vi "Generic Controller with DSA.vi"() -> ()   [LabVIEW 2017]
uses:
  <vilib>/myRIO/Instrument Drivers/Onboard IO/AO/typedefs/AO Reference.ctl
  <vilib>/myRIO/Common/Instrument Driver Framework/Utilities/typedefs/myRIO Generic Hardware Reference.ctl
  <vilib>/myRIO/Common/Instrument Driver Framework/Utilities/typedefs/Hardware Version Enum.ctl
  <vilib>/myRIO/Common/Instrument Driver Framework/Utilities/typedefs/myRIO v1.0 Reference.ctl
  <vilib>/myRIO/Common/Instrument Driver Framework/Utilities/typedefs/Generic FPGA Reference.ctl
  <vilib>/myRIO/Common/Instrument Driver Framework/myRIO v1.0/AO/typedefs/AO Channels List.ctl
  <vilib>/myRIO/Common/Instrument Driver Framework/myRIO v1.0/AO/typedefs/AO Channels Enum.ctl
  <vilib>/myRIO/Common/Instrument Driver Framework/Utilities/typedefs/Analog Scaling Constants List.ctl
  <vilib>/myRIO/Common/Instrument Driver Framework/Utilities/typedefs/Analog Scaling Constants.ctl
  <vilib>/userdefined/High Color/nirio_resource_hc.ctl
  <vilib>/Simulation/Scripting/Companion Diagram/SimConfigNode/SimParams.ctl
  <vilib>/Simulation/Scripting/Companion Diagram/SimConfigNode/_simSolvers.ctl
  <vilib>/Simulation/Implementation/Shared/SIMSCR Execution Mode.ctl
  <vilib>/Platform/TimedLoop/XDataNode/timing_clust.ctl
  <vilib>/Platform/TimedLoop/XDataNode/nitl_modes.ctl
  <vilib>/Platform/TimedLoop/XDataNode/wakeup.ctl
  <vilib>/Simulation/Param Hierarchy/Typedefs/SIMPH Param Control Actions.ctl
  <vilib>/Simulation/Implementation/Shared/SIM limit type.ctl
  <vilib>/Simulation/Scripting/Editor Utilities/SIM subVI tag data.ctl
  <vilib>/Simulation/Scripting/Editor Utilities/SIM subVI execution type.ctl
  <vilib>/myRIO/Instrument Drivers/Onboard IO/AI/typedefs/AI Reference.ctl
  <vilib>/myRIO/Common/Instrument Driver Framework/myRIO v1.0/AI/typedefs/AI Channels List.ctl
  <vilib>/myRIO/Common/Instrument Driver Framework/myRIO v1.0/AI/typedefs/AI Channels Enum.ctl
  <vilib>/myRIO/Common/Instrument Driver Framework/Utilities/vis/Is FPGA Ref Available.vi
  <vilib>/myRIO/Common/Instrument Driver Framework/myRIO v1.0/AO/vis/myRIO v1.1 Open AO.vi
  <vilib>/myRIO/Instrument Drivers/Onboard IO/AO/vis/Write.vi
  <vilib>/Simulation/Implementation/Shared/NILVSim_ParamChanged.vi
  <vilib>/Simulation/Implementation/Shared/NILVSim_FinishedLate.vi
  <vilib>/Simulation/Implementation/Shared/NILVSIM_BeginStep.vi
  <vilib>/myRIO/Common/Instrument Driver Framework/myRIO v1.0/AI/vis/myRIO v1.1 Open AI.vi
  <vilib>/myRIO/Instrument Drivers/Onboard IO/AI/vis/Read.vi
  <vilib>/Simulation/Utility/Implementation/SIM Halt.vi
  <vilib>/Simulation/DataSources/Implementation/NILVSim Signal Generator.llb/SIM Signal Generator (scalar).vi
  <vilib>/Simulation/Utility/Implementation/SIM SimulationParams.vi
  <vilib>/Simulation/ContinuousLinear/Implementation/NILVSim Integrator new.llb/SIM Integrator distributor (scalar).vi
  <vilib>/Simulation/Implementation/Shared/SIM Is Init or Final Stage.vi
  <vilib>/Simulation/Implementation/Shared/SIM Fire Discrete SubVI.vi
  <vilib>/Simulation/SignalArithmetic/Implementation/NILVSim Gain.llb/SIM Gain (scalar).vi
  <vilib>/Simulation/ContinuousLinear/Implementation/NILVSim Integrator new.llb/SIM Integrator collector (scalar).vi
  <vilib>/Simulation/ContinuousLinear/Implementation/NILVSim Transfer Function Direct.llb/SIM Transfer Function Direct (SISO).vi
  <vilib>/Simulation/Implementation/Shared/NILVSim_Manager.vi
  <vilib>/Utility/error.llb/Clear Errors.vi
  <vilib>/Simulation/Implementation/Shared/NILVSim_FinalizeModel.vi
  <vilib>/myRIO/Common/Instrument Driver Framework/Utilities/vis/Validate Channels.vi
  <vilib>/myRIO/Common/Instrument Driver Framework/myRIO v1.0/AO/vis/myRIO v1.0 Reserve AO.vi
  <vilib>/myRIO/Common/Instrument Driver Framework/myRIO v1.0/AI/vis/myRIO v1.0 Reserve AI.vi
  <vilib>/Simulation/Utility/Implementation/NILVSim SimulationParams (core).vi
  <vilib>/Simulation/Implementation/Shared/SIM Fire Discrete SubVI (Core).vi
  <vilib>/myRIO/Common/Instrument Driver Framework/myRIO v1.0/AO/vis/myRIO v1.0 Build MUX Configuration AO.vi
  <vilib>/myRIO/Common/Instrument Driver Framework/myRIO v1.0/Resource Manager/vis/myRIO v1.0 Reserve Channel List.vi
  <vilib>/myRIO/Common/Instrument Driver Framework/myRIO v1.0/AI/vis/myRIO v1.0 Build MUX Configuration AI.vi
  <vilib>/myRIO/Common/Instrument Driver Framework/myRIO v1.0/Resource Manager/vis/myRIO v1.0 Reserve Channel.vi
  <vilib>/myRIO/Common/Instrument Driver Framework/myRIO v1.0/Resource Manager/vis/myRIO v1.0 Unreserve Channel.vi
  <vilib>/myRIO/Common/Instrument Driver Framework/myRIO v1.0/Resource Manager/vis/myRIO v1.0 Build Mutex Name.vi
  <vilib>/Utility/VariantDataType/GetNumericInfo.vi
  <vilib>/Utility/error.llb/Error Cluster From Error Code.vi
  <vilib>/myRIO/Common/Instrument Driver Framework/myRIO v1.0/myRIO v1.1 Open.vi
  <vilib>/myRIO/Common/Instrument Driver Framework/myRIO v1.0/AO/vis/myRIO v1.0 Get Scaling Constants AO.vi
  <vilib>/myRIO/Common/Instrument Driver Framework/Utilities/vis/IO Manager.vi
  <vilib>/myRIO/Common/Instrument Driver Framework/Utilities/vis/Configuration Manager.vi
  <vilib>/myRIO/Common/Instrument Driver Framework/myRIO v1.0/myRIO v1.0 Close.vi
  <vilib>/myRIO/Common/Instrument Driver Framework/myRIO v1.0/AO/vis/myRIO v1.0 Write AO.vi
  <vilib>/Simulation/Implementation/Shared/SIM Unbundle Sim Info.vi
  <vilib>/Simulation/Implementation/Shared/SIMSH Read Queue.vi
  <vilib>/Simulation/Implementation/Shared/NILVSim_Initialize.vi
  <vilib>/myRIO/Common/Instrument Driver Framework/myRIO v1.0/AI/vis/myRIO v1.0 Get Scaling Constants AI.vi
  <vilib>/myRIO/Common/Instrument Driver Framework/myRIO v1.0/AI/vis/myRIO v1.0 Read AI.vi
  <vilib>/Simulation/Utility/Implementation/NILVSim Get Time and IsAcceptedStep.vi
  <vilib>/Simulation/Implementation/Shared/NILVSim_GetModelError.vi
  <vilib>/Simulation/Implementation/Shared/SIM Bundle Sim Info.vi
  <vilib>/myRIO/Express VI/Onboard IO/AO/AO Express VI.xnode
  <vilib>/myRIO/Instrument Drivers/Onboard IO/AO/vis/myRIO AO Open.xnode
  <vilib>/Platform/TimedLoop/XDataNode/XDataNode.xnode
  <vilib>/Simulation/Scripting/Companion Diagram/SimConfigNode/SimDog.xnode
  <vilib>/myRIO/Express VI/Onboard IO/AI/AI Express VI.xnode
  <vilib>/myRIO/Instrument Drivers/Onboard IO/AI/vis/myRIO AI Open.xnode
  <vilib>/Simulation/Implementation/XNodeFramework/SimXNode/SimX.xnode
  <vilib>/Simulation/ContinuousLinear/Implementation/NILVSim Integrator new.llb/SIM Integrator (scalar).vi
  <vilib>/myRIO/Instrument Drivers/Onboard IO/AO/AO.lvlib
  <vilib>/Platform/TimedLoop/XDataNode/XDNodeRunTimeDep.lvlib
  <vilib>/myRIO/Instrument Drivers/Onboard IO/AI/AI.lvlib
  <vilib>/Simulation/Implementation/Shared/NI_SIM_Implementation.lvlib
panel:
  in  "Tab Control":T1(tab)
  in  "alpha":dbl=10.0
  in  "Td":dbl=0.0025
  in  "ON? 2":bool=TRUE
  in  "Upper":dbl=10.0
  in  "Lower":dbl=-10.0
  in  "Ti":dbl=0.0032
  in  "ON?":bool
  in  "Kp":dbl=-6.1
  in  "Feedback?":bool=TRUE
  in  "Amplitude":dbl
  in  "Frequency":dbl=6.0
  in  "Offset":dbl=0.04
  in  "Signal Type":u16(ring) items=["Sine", "Square", "Sawtooth", "Random"]
  in  "Control Time Step [s]":dbl=0.0005
  out "Control Loop Execution Time [us]":u32=249
  out "Control Loop Late Cycles":i32=4
  in  "External Reference?":bool
  in  "Internal Reference?":bool
  out "Oscilliscope":T2(graph)={"Double"=0.0, "Double"=-0.429687544, "Double"=-2.605132217660948}
  out "Plot Loop Execution Time [us]":u32=565
  in  "TLP":dbl=0.0016
  in  "ON? 3":bool=TRUE
  out "DSA Loop Late Cycles":i32
  out "DSA Loop Execution Time (us)":u32=518
  out "Bode Phase":cluster{dbl[], dbl[]}(graph)={[0.5, 0.5413183669370273, 0.5860511487667401, 0.6344805015839611, 0.6869118979416314, 0.7436760536467557, 0.8051310137804697, 0.8716644110999939, 0.9436959110675486, 1.021679858928471, 1.1061081455352246, 1.1975133099937427, 1.2964718987023336, 1.4036081019705886, 1.5195976911565985, 1.6451722811563343, 1.781123945131221, 1.9283102105817356, 2.0876594682802008, 2.2601768281801213, 2.446950459238747, 2.649158453141854, 2.8680762552243393, 3.1050847094578082, 3.3616787682496687, 3.6394769219915744, 3.9402314078349554, 4.265839262086405, 4.618354285936929, 5.0], [1.1113686665475342, -3.3715278086255864, -4.589885860566625, 4.2977168391159495, -5.935917889942033, -4.065647863471284, -1.6158442409451226, 89.88669974540309, 70.62051910594798, 85.09208365468596, 77.00702996239605, 43.46670720052916, -2.679772948914234, -13.624983803961307, -15.540260691171454, 92.75050103936908, 65.66683642318564, 75.45823036346658, -6.144982127247204, -15.535633497005172, 63.51301466180453, -63.682873216459825, 64.9522046090478, -8.82711887868328, 21.07479668472711, 17.564687083801523, -3.3971444036905964, -1.5249224157625818, -0.7028110405561847, -10.27143238102737]}
  out "Bode Magnitude":cluster{dbl[], dbl[]}(graph)={[0.5, 0.5413183669370273, 0.5860511487667401, 0.6344805015839611, 0.6869118979416314, 0.7436760536467557, 0.8051310137804697, 0.8716644110999939, 0.9436959110675486, 1.021679858928471, 1.1061081455352246, 1.1975133099937427, 1.2964718987023336, 1.4036081019705886, 1.5195976911565985, 1.6451722811563343, 1.781123945131221, 1.9283102105817356, 2.0876594682802008, 2.2601768281801213, 2.446950459238747, 2.649158453141854, 2.8680762552243393, 3.1050847094578082, 3.3616787682496687, 3.6394769219915744, 3.9402314078349554, 4.265839262086405, 4.618354285936929, 5.0], [0.1705227721348142, 0.1544347188687134, 0.17822285984429972, 0.14890848479663207, 0.1556998177366923, 0.14229088999240103, 0.16278672493894716, 0.003754159491098782, 0.007278718638241219, 0.004240175333076675, 0.006838804760208183, 0.0620848402718586, 0.2688203440065051, 0.18402355770794834, 0.14230747948833408, 0.0022001806117035714, 0.003041606136419923, 0.004363980185748692, 0.14874482575873157, 0.16349358042061182, 0.014255687186903598, 0.18481000781841925, 0.01857244313127678, 0.16431673209279352, 0.212603582029145, 0.27808950044049247, 0.29698413361699644, 0.28891790694466224, 0.2871852670976697, 0.29582840306665104]}
  in  "START":bool
  out "Running":bool
  in  "Excitation Specs":T3={"Initial Frequency"=0.5, "Final Frequency"=5.0, "Number of Frequencies"=30, "DSA Samping Time [s]"=0.0005, "Amplitude"=0.01, "Offset"=0.0, "Freq Unit"=TRUE}
  in  "Cycle Specs":T4={"Cycles To Settle (M)"=1, "Cycles To Calculate (N)"=10}
  out "Stopped":bool=TRUE
  in  "STOP":bool
  out "Live Signals":cluster{"DSA Excitation":dbl, "output y(t)":dbl}(graph)={"DSA Excitation"=-2.605132217660948, "output y(t)"=-0.429687544}
  in  "Exit Program":bool
  # "PMCL Generic Controller with DSA"
  # "Control Loop Parameters"
  # "Reference Signal"
  # "Internal Reference"
  # "Controllers"
  # "Controllers Implemenetation"
  # "The Lead-Lag Controller has the form:"
  # "HF LP\nFilter:"
  # "Proportional:"
  # "Intergrator Limits"
  # "Lag:"
  # "Note: Ti is the integrator time constant. Ti = 1/Ki"
  # "Lead:"
  # "Note: Td is the lag compensator time constant."
  # "Note: Both references should be off when running the DSA!"
  # "Dynamic Signal Analyzer"
  # "Controls"
  # "Phase"
  # "Magnitude"
  # "Excitation Frequencies"
  # "Excitation Magnitude"
  # "Freq. Units"
  # "[Hz]"
  # "[rad/s]"
  # "Using the Controller\n \n(1) Press CNTRL + E to pull up the back pannel code.\n\n(2) Program your controller into the area labed:  \n\n(3) Check                             to enable your controller."
  # "Closed Loop Controller"
  # "Wiring Details\n  \n       - AO 0:   Control Effort\n \n       - AI   0+: Plant / Sensor Ouput\n       - AI   0- : AGND\n \n       - AI   1+: External Signal Generator \n       - AI   1- : AGND"
  # "- Ideally you would want AI 0+ to be the plant output. However as the plant output is not \n         always a voltage, this will often be a sensor output. As a result, the measured frequency \n         response (bode plots) will be gained by the gain of the sensor.\n \n              ~ Usually the gain of the sensor is a constant though so just divide the magnitude by it."
  # "Using the DSA\n \n(1) Press CNTRL + E to pull up the back pannel code.\n\n(2) Rewire                                        and                                        according to the TF you want to measure. See DSA Theory Tab for help.\n \n         TF = (DSA CH B) / (DSA CH B)  \n \n      - If using the DSA to measure a TF that's apart of the closed loop, make sure the closed loop is stable &                               .      \n \n(3) Turn off the reference signals:                                             &\n\n      - If using one of the reference signals to instead provide a DC bias, simply turn the amplitude to zero intead.\n\n(4) Set the DSA Excitation Specs & Cycel Specs: \n \n      - Inital Frequency: First frequnecy we want to measure. Typically atleast 1 decade before frequency of interest\n \n      - Final Frequency: Final frequency we want to measure. Typically atleast 1 decade beyond frequency of interest\n  \n             ~ Note:  Max Final Frequency = Sampling Rate/2     as this is out Nyquist Frequency          \n \n      - Number of Frequnecies: Something reasonable like 30 frequencies every decade measured\n \n      - Amplitude: Largest Amplitude such that the control effort does not staturate\n \n      - Cycles to Settle (M): 1 minimum for low frequencies (below 5 Hz) & 10 minimum for high frequencies (above 100 Hz)\n \n      - Cycles to Calculate (N): 1 minimum for low frequencies (below 5 Hz) & 100 minimum for high frequencies (above 100 Hz)  \n \n      * TO MAKE THE DSA FASTER WITH BETTER RESULTS, RUN THE DSA MULTIPLE TIMES!!! \n         ex. from     0.5 Hz - 5 Hz w/ M =1,    N =1, 5 Hz - 50 Hz w/ M = 1,  N = 10,     &    50 Hz - 500 Hz w/ M = 10, N = 100 \n \n(5) Press START to start the DSA.\n\n(6) Press STOP to stop the DSA if needed or it will stop when it is finished."
  # "Running the Program\n \n(1) Set the Controller Time Step, the rate at which the myRIO samples the sensor and updates the control effort sent to the plant.\n      This is located on the on the Controller Tab.\n\n      - Controller Loop Rate = 1/(Controller Time Step)     where the default is 0.001 sec which is a sampling rate of 1 kHz.\n \n      - If the Control Loop Late Cycles indicator rapidly increases, the control loop needs to run at a slower rate.\n \n      - If you update the Controller Time Step, exist and rerun the program! This must be set before the program starts.\n\n(2) If you plan on using the Dynamics Signal Anayzer to measure a frequency response, set the DSA Sampling Time [s], the rate at \n      which the dynamic signal analyzer samples the control signals at. This is located on the on the DSA Tab.\n\n      - DSA Sampling Rate = 1/(DSA Sampling Time)     where the default is 0.001 sec which is a sampling rate of 1 kHz.\n\n      - Typically, the  DSA Sampling Time =  Controller Time Step.\n \n      - Note: If the DSA Loop Late Cycles indicator rapidly increases, the DSA loop needs to run at a slower rate.\n \n      - If you update the Controller Sampling Time, exist and rerun the program! This must be set before the program starts.\n \n \n(2) Press the white arrow above,          , to start the program.\n \n(3) Use the program. See Using the Controller, Using the DSA, and/or Collecting Data.\n \n(4)  Click EXIT PROGRAM in the upper right hand corner to stop the progam. \n\n      - NEVER CLICK the small stop sign,          , unless it's an emergency as this will not reset your AOs to zero."
  # "Collecting Data\n \n(1) Right click the graph and select Export.\n \n      - NOTE: You can only record what is shown on the graph!\n\n(2) Choose the format you want to export your data to:\n \n       - Export Data To Clipboard: Copies it so you can paste it into a program like Excel, Matlab, Notepad, etc.\n \n       - Export Data To Excel: Opens up your data in Excel.\n \n       - Export Simpliefed Image... : Saves your data as a cleaned up screenshot picture\n  \n Changing the Total Time of Data Recorded\n \nTo change the length of time displayed on the graph and thus the length of time you record data for, right click and select Chart History Length while the porgram is NOT running. \n \n        Chart History Length = [ (Desired Length of Time in Sec) / (Controller Time Step) ] + 1\n \n        * The + 1 is necessary to prevent the axes from drifting as LabVIEW includes both the start and final sample in the total time.\n\nThen double click on the starting and final tick of the time axis. Type a new a time into each tick such that the total time elapsed between the two ticks is your desired length of time to be displayed."
  # "A DSA, or Dynamic Signal Analyzer is a tool that measures a the frequency response of a transfer function and plots its corresponding bode plots."
  # "A DSA works in 3 steps:\n\n      (1) The DSA  inputs a swept sine wave (a sine wave that increaes in frequency), D, into the control loop. Here the swept sine wave is being added to the reference at the feedback summing junction. The swept sine wave will show up through out the control loop with different a \n            magnitude and phase at each of its frequencies. How the magnitude and phase of this swept sine wave changes at each frequency through out the control loop is what we care about.\n\n      (2) Then the DSA measures the swept sine wave at two points through out the control loop.\n\n      (3) Finally the DSA finds the frequency response of the  transfer function between the two points measured. This is visually shown as a bode plot. \n            \n                  - The  magnitude of the frequency response is the magnitude of the swept sine wave measured at the first point divided the  magnitude of the swept sine wave measured at the second point. \n\n                  - The phase of the frequency response is the phase of the swept sine wave measured at the first point minus the phase of the swept sine wave measured at the second point.\n\nThree transfer functions we often care about are the plant P, return ratio RR, and the closed loop CL. Thus below we will go through how to measure the frequency response of those with the DSA.\n\n      - Plant: The plant is just the ratio of the output of the plant to its input, P = Y/C. Thus the DSA finds the frequency response of the plant by measuring the signal output by the plant (a swept sine wave), Y, and the signal input to the plant (a swept sine wave), C. Then it divides \n                    the magnitude of Y by the magnitude of C and subtracts the phase of C from the phase of Y at each frequency of the swept sine wave. This provides the frequency reponse of the plant as it changes with freqency.\n\n      - Return Ratio: The return ratio is just the ratio of the output of the loop to its input, RR = M/E. Thus the DSA finds the frequency response of the return ratio by measuring the signal output by the loop (a swept sine wave), M, and the signal input to the loop (a swept sine wave), E. \n                                 Then it divides the magnitude of M by the magnitude of E and subtracts the phase of E from the phase of M at each frequency of the swept sine wave. This provides the frequency reponse of the return ratio as it changes with freqency.\n\n      - Closed Loop: The closed loop is just the ratio of the output of the closed loop to its input, CL = Y/D. Thus the DSA finds the frequency response of the closed loop by measuring the signal output by the closed loop (a swept sine  wave), Y, and the signal input to the closed loop \n                                 (a swept sine wave), D. Then it divides the magnitude of Y by the magnitude of D and subtracts the phase of R from the phase of Y at each frequency of the swept sine wave. This provides the frequency reponse of the closed loop as it changes with freqency."
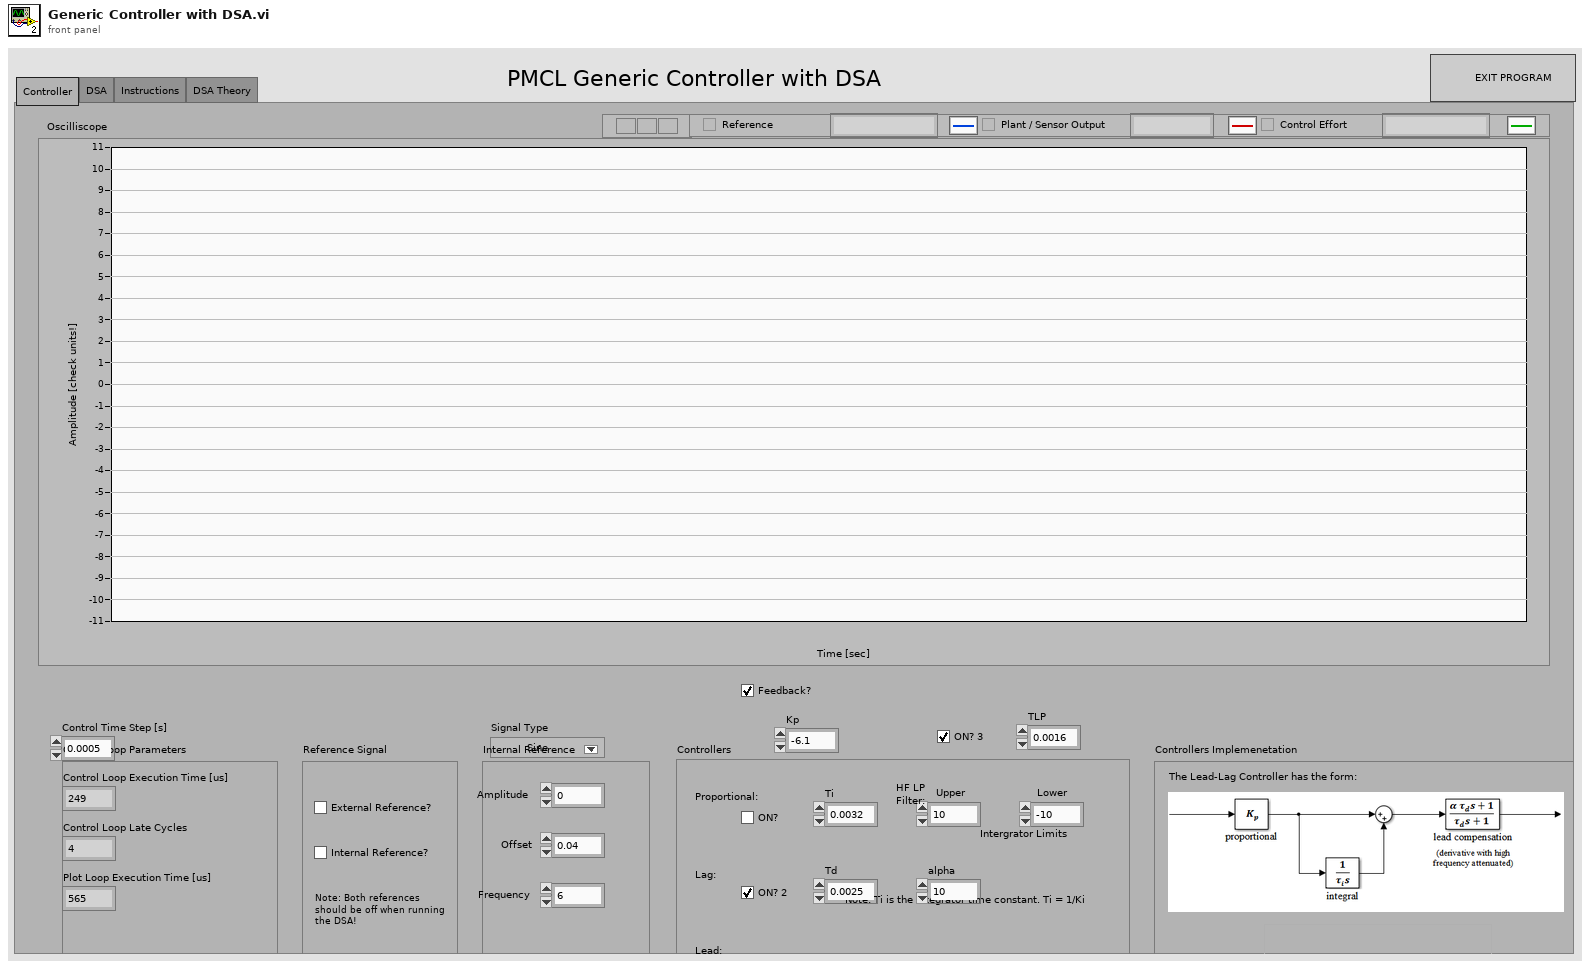
[diagram p1: front panel]
types:
  T1 = enum32{"Controller", "DSA", "Instructions", "DSA Theory"}
  T2 = cluster{"Double":dbl, "Double":dbl, "Double":dbl}
  T3 = cluster{"Initial Frequency":dbl, "Final Frequency":dbl, "Number of Frequencies":i16, "DSA Samping Time [s]":dbl, "Amplitude":dbl, "Offset":dbl, "Freq Unit":bool}
  T4 = cluster{"Cycles To Settle (M)":i16, "Cycles To Calculate (N)":i16}
  T5 = cluster{"DSA Excitation":dbl, "output y(t)":dbl}[]
  T6 = cluster{"Double":dbl, "Double":dbl, "Double":dbl}[]
  T7 = typedef "AO.lvlib/AO Reference.ctl" = cluster{"myRIO Reference":T8, "AO Channel List":T12, "AO Scaling Constant List":T14}
  T8 = typedef "myRIO Generic Hardware Reference.ctl" = cluster{"myRIO Model":T9, "myRIO Hardware Reference":T10}
  T9 = typedef "Hardware Version Enum.ctl" = enum16{"Unknown", "myRIO-1900", "myRIO-1950", "roboRIO", "NI ELVIS RIO CM"}
  T10 = typedef "myRIO v1.0 Reference.ctl" = cluster{"Generic FPGA Reference":T11, "Allow multiple opens":bool}
  T11 = typedef "Generic FPGA Reference.ctl" = refnum<k20>
  T12 = typedef "AO Channels List.ctl" = T13[]
  T13 = typedef "AO Channels Enum.ctl" = enum16{"Not Connected", "AudioOut/Left", "AudioOut/Right", "C/AO0", "C/AO1", "A/AO0", "A/AO1", "B/AO0", "B/AO1"}
  T14 = typedef "Analog Scaling Constants List.ctl" = T15[]
  T15 = typedef "Analog Scaling Constants.ctl" = cluster{"LSB Weight (Volts)":dbl, "Offset (Volts)":dbl, "Signed?":bool}
  T16 = typedef "nirio_resource_hc.ctl" = tag
  T17 = typedef "XDNodeRunTimeDep.lvlib/timing_clust.ctl" = cluster{"Expected End [f-1]":u64, "Actual End [f-1]":u64, "Finished Late? [f-1]":bool, "Expected End [i-1]":u64, "Actual End [i-1]":u64, "Finished Late? [i-1]":bool, "Expected Start [i]":u64, "Actual Start [i]":u64, "Expected Start [f]":u64, "Actual Start [f]":u64, "Source Name":string, "Structure Name":string, "Period":i64, "Deadline":i64, "Offset":i64, "Start":i64, "Priority":i32, "Timeout":i32, "Mode":T18, "Wakeup Reason":T19, "Error":errorcluster, "Source Type":string, "Secondary Source Type":string, "Global End Time":u64, "Global Start Time":u64, "Frame Duration":u64, "Iteration Duration":u64, "Assigned CPU":i32, "I/O Scan Engine Mode":u32}
  T18 = typedef "XDNodeRunTimeDep.lvlib/nitl_modes.ctl" = enum32{"No Change", "Process missed periods, maintain original phase", "Discard missed periods, maintain original phase", "Process missed periods, ignore original phase", "Discard missed periods, ignore original phase"}
  T19 = typedef "XDNodeRunTimeDep.lvlib/wakeup.ctl" = enum32{"Normal", "Aborted", "Asynchronous wakeup", "Timing source error", "Timed loop error", "Timeout"}
  T20 = typedef "SimParams.ctl" = cluster{"Initial Time (s)":dbl, "Final Time (s)":dbl, "Step Size (s)":dbl, "ODE Solver":T21, "Minimum Step Size (s)":dbl, "Maximum Step Size (s)":dbl, "Relative Tolerance":dbl, "Absolute Tolerance":dbl, "Software Timing":bool, "Initial Step Size (s)":dbl, "Automatic Fixed Step Size?":bool, "Automatic Discrete Step Size?":bool, "Discrete Step Size (s)":dbl, "Calculate using Time Step":bool, "Solver Wired?":bool, "Prev.Frm.Expected End":u64, "Prev.Frm.Actual End":u64, "Prev.Frm.Finished Late?":bool, "Prev.Iter.Expected End":u64, "Prev.Iter.Actual End":u64, "Prev.Iter.Finished Late?":bool, "Expected Iteration Start":u64, "Actual Iteration Start":u64, "Expected Frame Start":u64, "Actual Frame Start":u64, "Source Name":string, "Name":string, "Period":i64, "Deadline":i64, "Offset":i64, "Start":i64, "Priority":i32, "Timeout":i32, "Processor":i32, "Mode":enum32{"No Change", "Process missed periods, maintain original phase", "Discard missed periods, maintain original phase", "Process missed periods, ignore original phase", "Discard missed periods, ignore original phase"}, "Wakeup reason":enum32{"Normal", "Aborted", "Asynchronous wakeup", "Timing source error", "Timed loop error", "Timeout"}, "Error":errorcluster, "Source Type":string, "Secondary Source Type":string, "Global End Time":u64, "Global Start Time":u64, "Full Solver Reset":bool, "Execution Mode":T22, "Nan/Inf Check":bool, "Custom Solver Library":string, "Solver Is Variable":bool, "custom solver name":string, "Signal Collection Decimation":u32}
  T21 = typedef "_simSolvers.ctl" = enum16{"Runge-Kutta 1 (Euler)", "Runge-Kutta 2", "Runge-Kutta 3", "Runge-Kutta 4", "Runge-Kutta 23 (variable)", "Runge-Kutta 45 (variable)", "BDF (variable)", "Adams-Moulton (variable)", "Rosenbrock (variable)", "Discrete States Only", "SDIRK 4 (variable)", "Radau 5 (variable)", "Radau 9 (variable)", "Radau 13 (variable)", "Radau [Variable Order] (variable)", "Gear's Method (variable)", "Linearizer", "State Query", "Trim Eval", "Custom Solver"}
  T22 = typedef "SIMSCR Execution Mode.ctl" = enum16{"Simulate to Completion", "Single Time-Step Simulation (Fixed Step Only)"}
  T23 = typedef "AI.lvlib/AI Reference.ctl" = cluster{"myRIO Reference":T8, "AI Channels List":T24, "AI Scaling Constants List":T14}
  T24 = typedef "AI Channels List.ctl" = T25[]
  T25 = typedef "AI Channels Enum.ctl" = enum16{"Not Connected", "AudioIn/Left", "AudioIn/Right", "C/AI0", "C/AI1", "A/AI0", "A/AI1", "A/AI2", "A/AI3", "B/AI0", "B/AI1", "B/AI2", "B/AI3", "AI/AI0", "AI/AI1", "AI/AI2", "AI/AI3"}
  T26 = typedef "SIMPH Param Control Actions.ctl" = enum16{"get params", "set params"}
  T27 = typedef "SIM subVI tag data.ctl" = cluster{"period":dbl, "skew":dbl, "Simulation execution type":T28}
  T28 = typedef "SIM subVI execution type.ctl" = enum16{"Function call", "Discrete", "Continuous", "Initialization only", "Final step only"}
  T29 = typedef "SIM limit type.ctl" = enum16{"upper", "lower", "both", "none"}
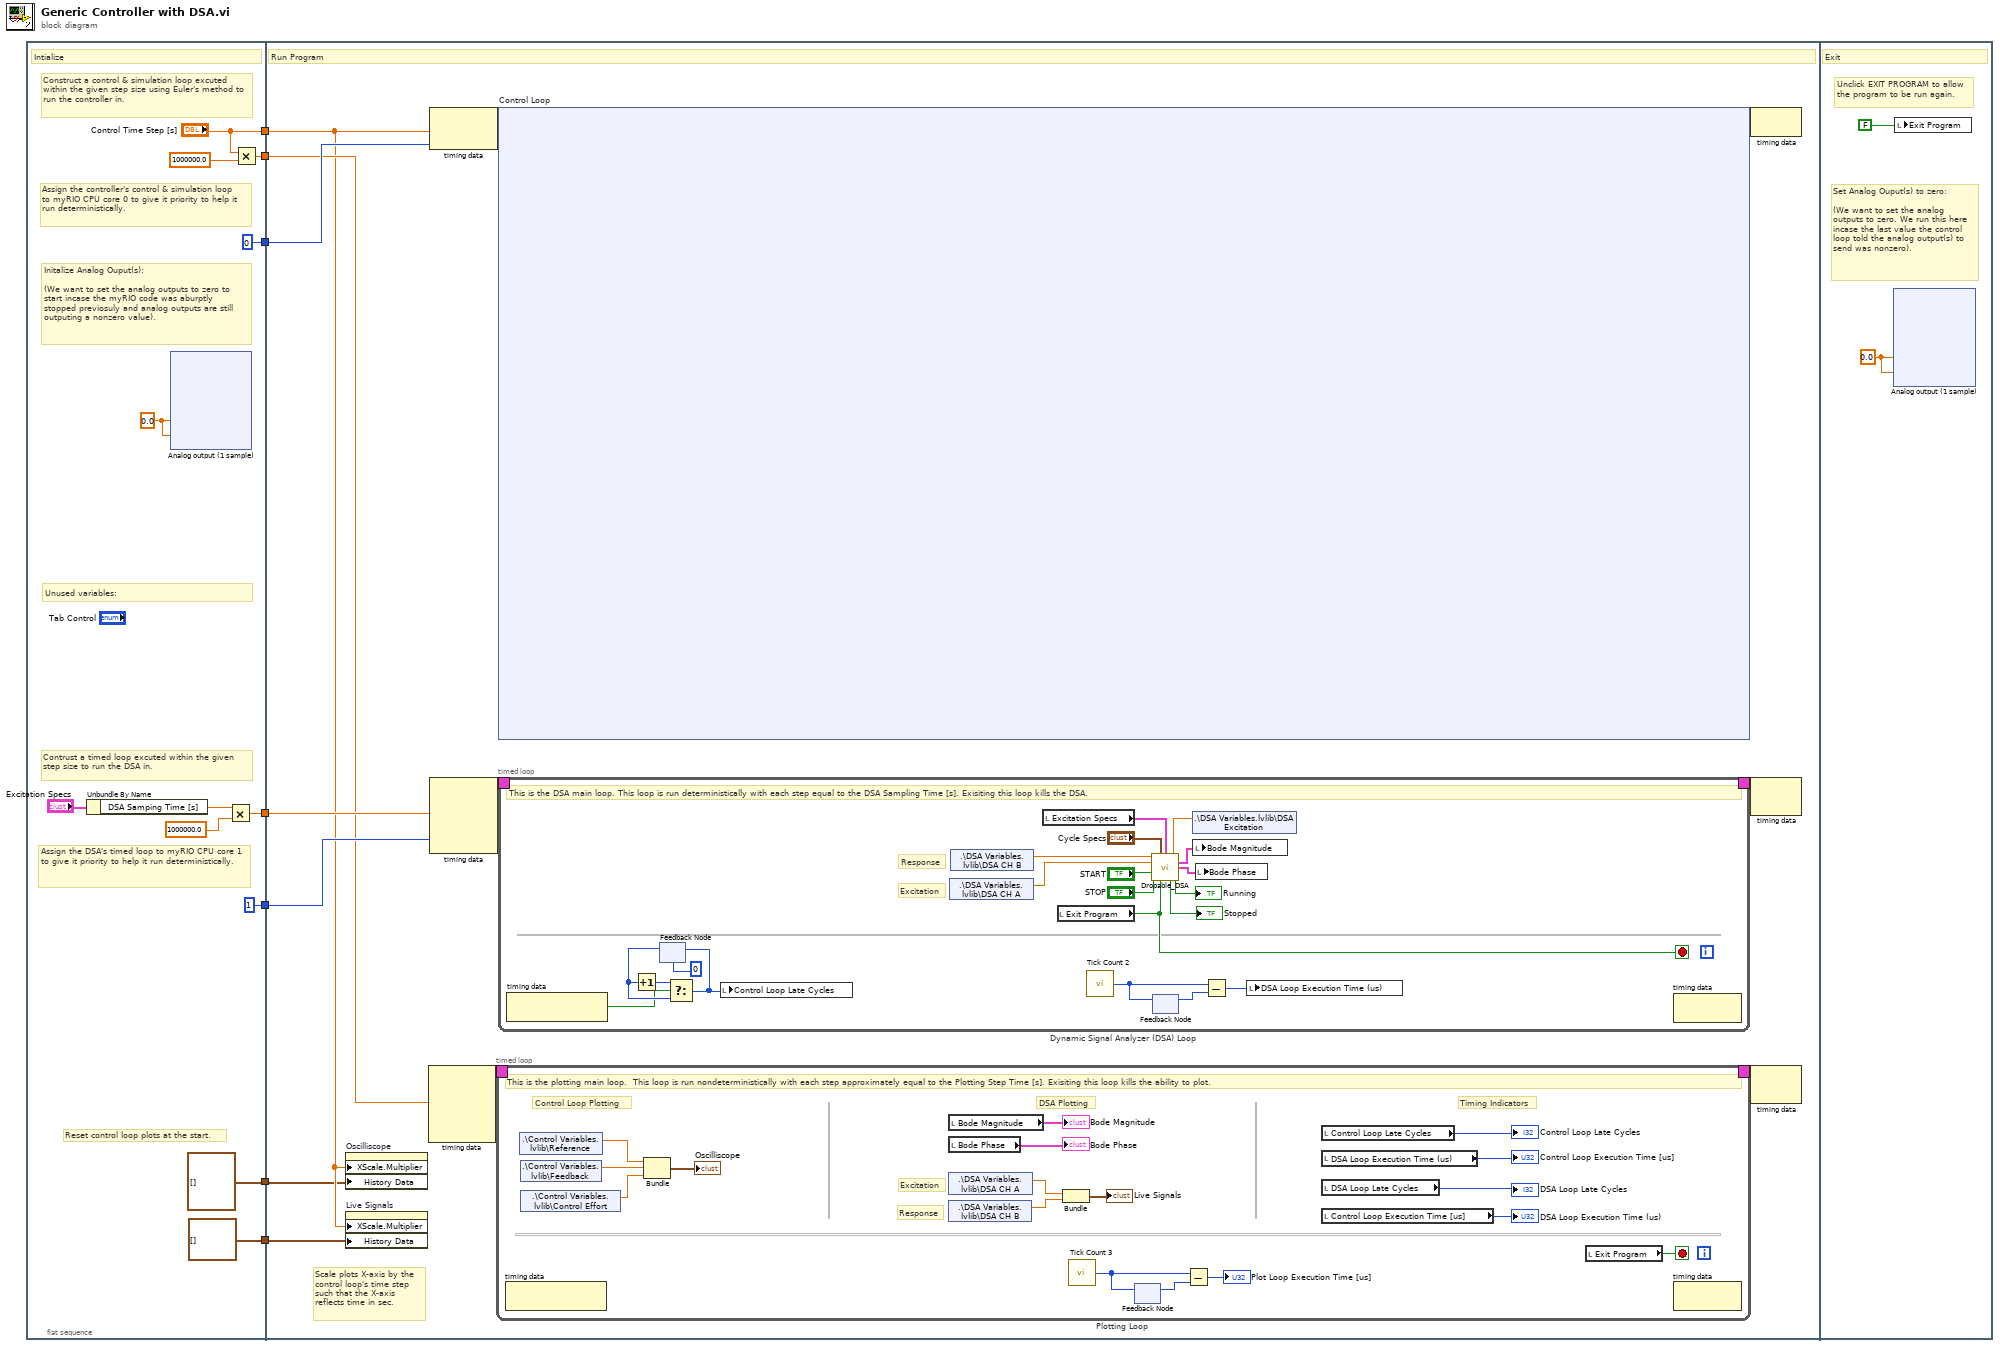
[diagram p0: block diagram]
diagram:
  n1 = flat-sequence {
    tunnel: ["Control Time Step [s]"] -> w7
    tunnel: [0 ("Processor")] -> w6
    tunnel: [w15] -> w5
    tunnel: [1 ("Processor")] -> w4
    tunnel: [w11] -> w3
    tunnel: [T6 [] ("History Data")] -> w2
    tunnel: [T5 [] ("History Data")] -> w1
    tunnel: w7 -> [w60]
    tunnel: w6 -> [w66]
    tunnel: w5 -> [w65]
    tunnel: w4 -> [w64]
    tunnel: w3 -> [w61]
    tunnel: w2 -> [w59]
    tunnel: w1 -> [w58]
    frame #0 {
      w10 = 0.0
      # "Reset control loop plots at the start."
      # "Assign the DSA's timed loop to myRIO CPU core 1 to give it priority to help it run deterministically."
      # "Contrust a timed loop excuted within the given step size to run the DSA in."
      # "Assign the controller's control & simulation loop to myRIO CPU core 0 to give it priority to help it run deterministically."
      # "Construct a control & simulation loop excuted within the given step size using Euler's method to run the controller in."
      # "Initalize Analog Ouput(s):\n\n(We want to set the analog outputs to zero to start incase the myRIO code was aburptly stopped previosuly and analog outputs are still outputing a nonzero value)."
      # "Unused variables:"
      # "Intialize"
      n2 = Unbundle By Name("Excitation Specs") -> ("DSA Samping Time [s]"=w16:dbl)
      n3 = xnode "Analog output (1 sample)"("Control Effort (C/AO0 (AO0))"=w10, "Signal To Probe (C/AO1 (AO1))"=w10) -> ()  [unwired: 1 in, 1 out]
      n4 = Multiply(x=w16, y=1000000.0) -> (x*y=w15:dbl)
      n5 = Multiply(x="Control Time Step [s]", y=1000000.0) -> (x*y=w11:dbl)
    }
    frame #1 {
      # "Scale plots X-axis by the control loop's time step such that the X-axis reflects time in sec."
      # "Run Program"
      n6 = property on="Oscilliscope" class="WFChart (strict)"("XScale.Multiplier"=w60, "History Data"=w59) -> ()  [unwired: 2 in, 2 out]
      n7 = property on="Live Signals" class="WFChart (strict)"("XScale.Multiplier"=w60, "History Data"=w58) -> ()  [unwired: 2 in, 2 out]
      n8 = node-c288(w61) -> (w63:T17)  [unwired: 3 in]
      n9 = node-c288(w60, w66) -> (w70:variant)
      n10 = node-c288(w65, w64) -> (w68:T17)  [unwired: 2 in]
      n11 = timed-loop "Plotting Loop" {
        timing: w63 -> [_]
        timing-out: [_] -> w62
        stop <- w87 stop-if-true
        # "Timing Indicators"
        # "DSA Plotting"
        # "Control Loop Plotting"
        # "Response"
        # "Excitation"
        # "This is the plotting main loop.  This loop is run nondeterministically with each step approximately equal to the Plotting Step Time [s]. Exisiting this loop kills the ability to plot."
        n12 = node-c288() -> ()  [unwired: 1 in, 1 out]
        n13 = shared-variable ".\\Control Variables.lvlib\\Reference"() -> (w75:dbl)  [unwired: 1 in, 1 out]
        n14 = shared-variable ".\\Control Variables.lvlib\\Feedback"() -> (w74:dbl)  [unwired: 1 in, 1 out]
        n15 = shared-variable ".\\Control Variables.lvlib\\Control Effort"() -> (w73:dbl)  [unwired: 1 in, 1 out]
        n16 = Bundle("Double"=w75, "Double"=w74, "Double"=w73) -> (→"Oscilliscope":T2)  [unwired: 1 in]
        n17 = local read "Bode Magnitude"() -> (→"Bode Magnitude":cluster{dbl[], dbl[]})
        n18 = local read "Bode Phase"() -> (→"Bode Phase":cluster{dbl[], dbl[]})
        n19 = shared-variable ".\\DSA Variables.lvlib\\DSA CH A"() -> (w71:dbl)  [unwired: 1 in, 1 out]
        n20 = shared-variable ".\\DSA Variables.lvlib\\DSA CH B"() -> (w72:dbl)  [unwired: 1 in, 1 out]
        n21 = Bundle("Double"=w71, "Double"=w72) -> (→"Live Signals":cluster{"Double":dbl, "Double":dbl})  [unwired: 1 in]
        n22 = call "Tick Count 3"() -> ("Tick Count(uSec)"=w82:u32)
        n23 = feedback #1() -> (w83:u32)  [unwired: 1 in]
        n24 = feedback-in #1 ("2")(w82) -> ()
        n25 = Subtract(x=w82, y=w83) -> (x-y=→"Plot Loop Execution Time [us]":u32)
        n26 = local read "Control Loop Late Cycles"() -> (→"Control Loop Late Cycles":i32)
        n27 = local read "DSA Loop Execution Time (us)"() -> (→"Control Loop Execution Time [us]":u32)
        n28 = local read "DSA Loop Late Cycles"() -> (→"DSA Loop Late Cycles":i32)
        n29 = local read "Control Loop Execution Time [us]"() -> (→"DSA Loop Execution Time (us)":u32)
        n30 = local read "Exit Program"() -> (w87:bool)
        n31 = node-c288() -> ()  [unwired: 1 in, 1 out]
      }
      n32 = node-c254 "Control Loop"(w70) -> (w69:variant)
      n33 = timed-loop "Dynamic Signal Analyzer (DSA) Loop" {
        timing: w68 -> [_]
        timing-out: [_] -> w67
        stop <- w102 stop-if-true
        # "Excitation"
        # "Response"
        # "This is the DSA main loop. This loop is run deterministically with each step equal to the DSA Sampling Time [s]. Exisiting this loop kills the DSA."
        n34 = node-c288() -> (w95:bool)  [unwired: 1 in]
        n35 = feedback #2 ("Feedback Node 2")(0 ("Constant 8")) -> (w97:i32)
        n36 = Increment(x=w97) -> (x+1=w96:i32)
        n37 = Select ("Select 4")(t=w96, s=w95, f=w97) -> (s? t:f=w99:i32)
        n38 = feedback-in #2 ("3")(w99) -> ()
        n39 = local write "Control Loop Late Cycles"(w99) -> ()
        n40 = shared-variable ".\\DSA Variables.lvlib\\DSA CH A"() -> (w93:dbl)  [unwired: 1 in, 1 out]
        n41 = shared-variable ".\\DSA Variables.lvlib\\DSA CH B"() -> (w112:dbl)  [unwired: 1 in, 1 out]
        n42 = local read "Excitation Specs"() -> (w111:T3)
        n43 = local read "Exit Program"() -> (w102:bool)
        n44 = call "Tick Count 2"() -> ("Tick Count(uSec)"=w100:u32)
        n45 = call "Dropable_DSA.vi"("TF Out (CH B)"=w112, "Cycle Specs"="Cycle Specs", "Excitation Specs"=w111, "TF In (CH A)"=w93, "START"="START", "STOP"="STOP", "Exist Porgram"=w102) -> ("Disturbance"=w105:dbl, "Bode Magnitude"=w104:cluster{dbl[], dbl[]}, "Bode Phase"=w103:cluster{dbl[], dbl[]}, "Stopped"=→"Stopped":bool, "Running"=→"Running":bool)  [unwired: 3 in, 1 out]
        n46 = feedback #3() -> (w101:u32)  [unwired: 1 in]
        n47 = feedback-in #3 ("2")(w100) -> ()
        n48 = shared-variable ".\\DSA Variables.lvlib\\DSA Excitation"(w105) -> ()  [unwired: 1 in, 1 out]
        n49 = local write "Bode Magnitude"(w104) -> ()
        n50 = local write "Bode Phase"(w103) -> ()
        n51 = Subtract(x=w100, y=w101) -> (x-y=w94:u32)
        n52 = local write "DSA Loop Execution Time (us)"(w94) -> ()
        n53 = node-c288() -> ()  [unwired: 1 in, 1 out]
      }
      n54 = node-c288(w69) -> ()  [unwired: 1 out]
      n55 = node-c288(w67) -> ()  [unwired: 1 out]
      n56 = node-c288(w62) -> ()  [unwired: 1 out]
    }
    frame #2 {
      w1012 = 0.0
      # "Unclick EXIT PROGRAM to allow the program to be run again."
      # "Set Analog Ouput(s) to zero:\n\n(We want to set the analog outputs to zero. We run this here incase the last value the control loop told the analog output(s) to send was nonzero)."
      # "Exit"
      n57 = xnode "Analog output (1 sample)"("Control Effort (C/AO0 (AO0))"=w1012, "Signal to Probe (C/AO1 (AO1))"=w1012) -> ()  [unwired: 1 in, 1 out]
      n58 = local write "Exit Program"(FALSE) -> ()
    }
  }
